vi "Swerve Math.vi"(0 "Yaw":dbl=88.3, 2 "Rot. Point X":dbl, 3 "Rot. Point Y":dbl) -> (9 "Swerve Math Output":T1)   [LabVIEW 2019]
uses:
  Globals/Drive Train Global.vi
  Robot Information Global.vi
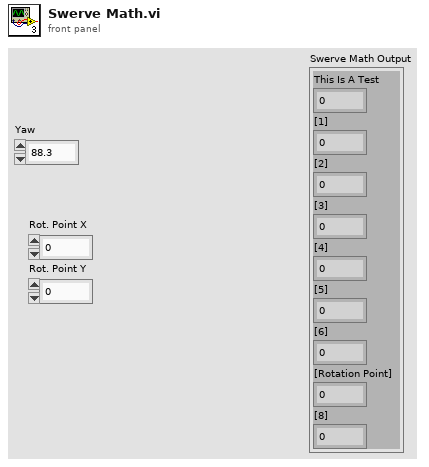
[diagram p1: front panel]
types:
  T1 = cluster{"This Is A Test":dbl, "[1]":dbl, "[2]":dbl, "[3]":dbl, "[4]":dbl, "[5]":dbl, "[6]":dbl, "[Rotation Point]":dbl, "[8]":dbl}
  T2 = cluster{"[0]":dbl, "[1]":dbl, "[2]":dbl, "[3]":dbl, "[4]":dbl, "[5]":dbl, "[6]":dbl, "[7]":dbl, "[8]":dbl}
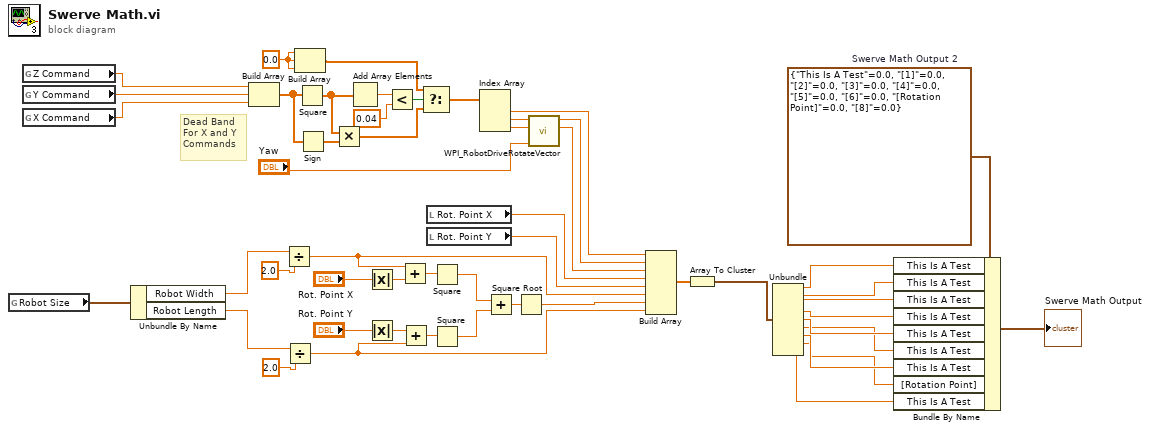
[diagram p0: block diagram]
diagram:
  w2 = T1 {"This Is A Test"=0.0, "[1]"=0.0, "[2]"=0.0, "[3]"=0.0, "[4]"=0.0, "[5]"=0.0, "[6]"=0.0, "[Rotation Point]"=0.0, "[8]"=0.0}  # Swerve Math Output 2
  w22 = 0.0 ("element")
  # "Dead Band \nFor X and Y\nCommands"
  n1 = global read "Robot Information Global.vi" "Robot Size"() -> (w29:cluster{"Robot Width":dbl, "Robot Length":dbl})
  n2 = global read "Drive Train Global.vi" "Z Command"() -> (w1:dbl)
  n3 = global read "Drive Train Global.vi" "Y Command"() -> (w17:dbl)
  n4 = global read "Drive Train Global.vi" "X Command"() -> (w30:dbl)
  n5 = Unbundle By Name(w29) -> ("Robot Width"=w27:dbl, "Robot Length"=w28:dbl)
  n6 = Build Array(w1, w17, w30) -> (w18:dbl[])
  n7 = Divide(x=w27, y=2.0) -> (x/y=w37:dbl)
  n8 = Divide(x=w28, y=2.0) -> (x/y=w15:dbl)
  n9 = Build Array(w22, w22, w22) -> (w23:dbl[])
  n10 = Square(x=w18) -> (x^2=w20:dbl[])
  n11 = Sign(1:w18) -> (0:w21:dbl[])
  n12 = Multiply(x=w20, y=w21) -> (x*y=w19:dbl[])
  n13 = Add Array Elements(numeric array=w20) -> (sum=w26:dbl)
  n14 = Absolute Value(x="Rot. Point X") -> (abs(x)=w51:dbl)
  n15 = Absolute Value(x="Rot. Point Y") -> (abs(x)=w49:dbl)
  n16 = Less?(x=w26, y=0.04 ("x")) -> (x < y?=w24:bool)
  n17 = Add(x=w37, y=w51) -> (x+y=w50:dbl)
  n18 = Add(x=w49, y=w15) -> (x+y=w48:dbl)
  n19 = Select(t=w23, s=w24, f=w19) -> (s? t:f=w34:dbl[])
  n20 = local read "Rot. Point X"() -> (w39:dbl)
  n21 = local read "Rot. Point Y"() -> (w38:dbl)
  n22 = Square(x=w50) -> (x^2=w46:dbl)
  n23 = Square(x=w48) -> (x^2=w47:dbl)
  n24 = Index Array(array=w34) -> (element #1=w32:dbl, element #2=w35:dbl, element #3=w40:dbl)  [unwired: 3 in]
  n25 = Add(x=w46, y=w47) -> (x+y=w45:dbl)
  n26 = Square Root(x=w45) -> (sqrt(x)=w36:dbl)
  n27 = call <vilib>:"WPI_RobotDriveRotateVector.vi"("Angle"="Yaw", "X"=w40, "Y"=w35) -> ("X'"=w33:dbl, "Y'"=w31:dbl)  [unwired: 7 out]
  n28 = Build Array(w32, w31, w33, w39, w38, w37, w36, w15) -> (w14:dbl[])
  n29 = Array To Cluster(array=w14) -> (cluster=w4:T2)
  n30 = Unbundle(w4) -> ("[0]"=w13:dbl, "[1]"=w12:dbl, "[2]"=w11:dbl, "[3]"=w10:dbl, "[4]"=w9:dbl, "[5]"=w8:dbl, "[6]"=w7:dbl, "[7]"=w6:dbl, "[8]"=w5:dbl)
  n31 = Bundle By Name(cluster=w2, "This Is A Test"=w13, "This Is A Test"=w12, "This Is A Test"=w11, "This Is A Test"=w10, "This Is A Test"=w9, "This Is A Test"=w8, "This Is A Test"=w7, "[Rotation Point]"=w6, "This Is A Test"=w5) -> (→"Swerve Math Output":T1)
